vi "VALEW_Sensors_Arc.vi"(0 "GEA2 Reference In":refnum<k24>, 1 "Number of Pulses":i32=6, 2 "Expected Degree Change":u16=360, 5 "GEA Inputs":T1={"Source"=228, "Destination"=35} {"Destination" format="%.0x"; "Source" format="%.0x"}, 7 "DAQmx Physical Channel":tag="9401_1/ctr2", 9 "Counter Terminal":tag="/9401_1/PFI4", 11 "Error In":errorcluster, 14 "Standalone?":bool=TRUE) -> (4 "GEA2 Reference Out":refnum<k24>, 6 "Pass/Fail?":bool, 8 "Report Text":string, 10 "Actual Degree Change":u16, 15 "Error Out":errorcluster)   [LabVIEW 2016, in "TLMB.lvlib"]
doc: "This VI generates clock ticks on the hall sensor and ensures that they increase the arc sensor ERD appropriately. 8 Ticks should equal 360 degrees"
uses:
  Projects/TLMB.lvlib
  Q:/Common/DLLs/GEA3/GeaCommunication.dll
  Common/DLLs/GEA3/GeaCommunication.dll
  Common/LabVIEW GEA2 Toolkit/LabVIEW_GEA2_Toolkit.lvlibp/type defs/Source_Destination.ctl
  Common/LabVIEW GEA2 Toolkit/LabVIEW_GEA2_Toolkit.lvlibp/type defs/ERD Read Data In.ctl
  Common/LabVIEW GEA2 Toolkit/LabVIEW_GEA2_Toolkit.lvlibp/type defs/Data Type.ctl
  <vilib>/DAQmx/create/channels.llb/DAQmx Create Channel (CO-Pulse Generation-Frequency).vi
  <vilib>/DAQmx/configure/timing.llb/DAQmx Timing (Implicit).vi
  Common/LabVIEW GEA2 Toolkit/LabVIEW_GEA2_Toolkit.lvlibp
  <resource>/objmgr/daqmx.rc
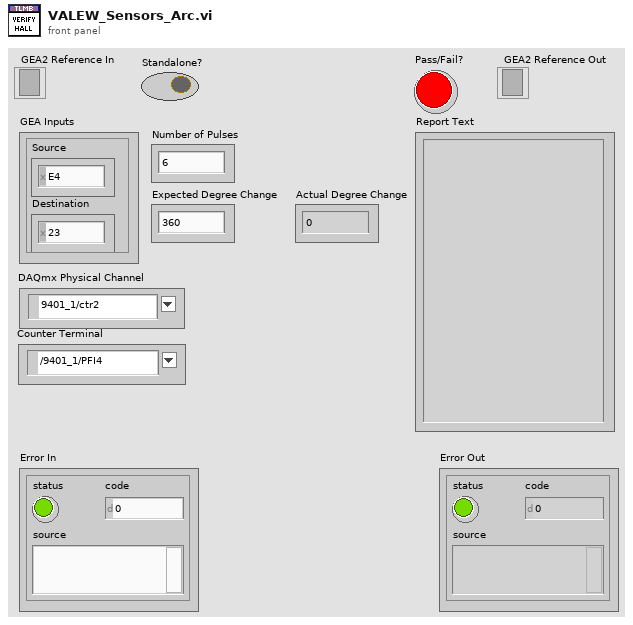
[diagram p1: front panel]
types:
  T1 = typedef "LabVIEW_GEA2_Toolkit.lvlibp/Source_Destination.ctl" = cluster{"Source":u8, "Destination":u8}
  T2 = typedef "LabVIEW_GEA2_Toolkit.lvlibp/ERD Read Data In.ctl" = cluster{"ERD Number":u16, "Data Type":T3}
  T3 = typedef "LabVIEW_GEA2_Toolkit.lvlibp/Data Type.ctl" = enum16{"string", "boolean", "uint8_t", "uint16_t", "uint32_t", "uint64_t", "int8_t", "int16_t", "int32_t", "int64_t"}
  T4 = typedef "LabVIEW_GEA2_Toolkit.lvlibp/ERD Read Data Out.ctl" = cluster{"ERD Number":u16, "Data":string}
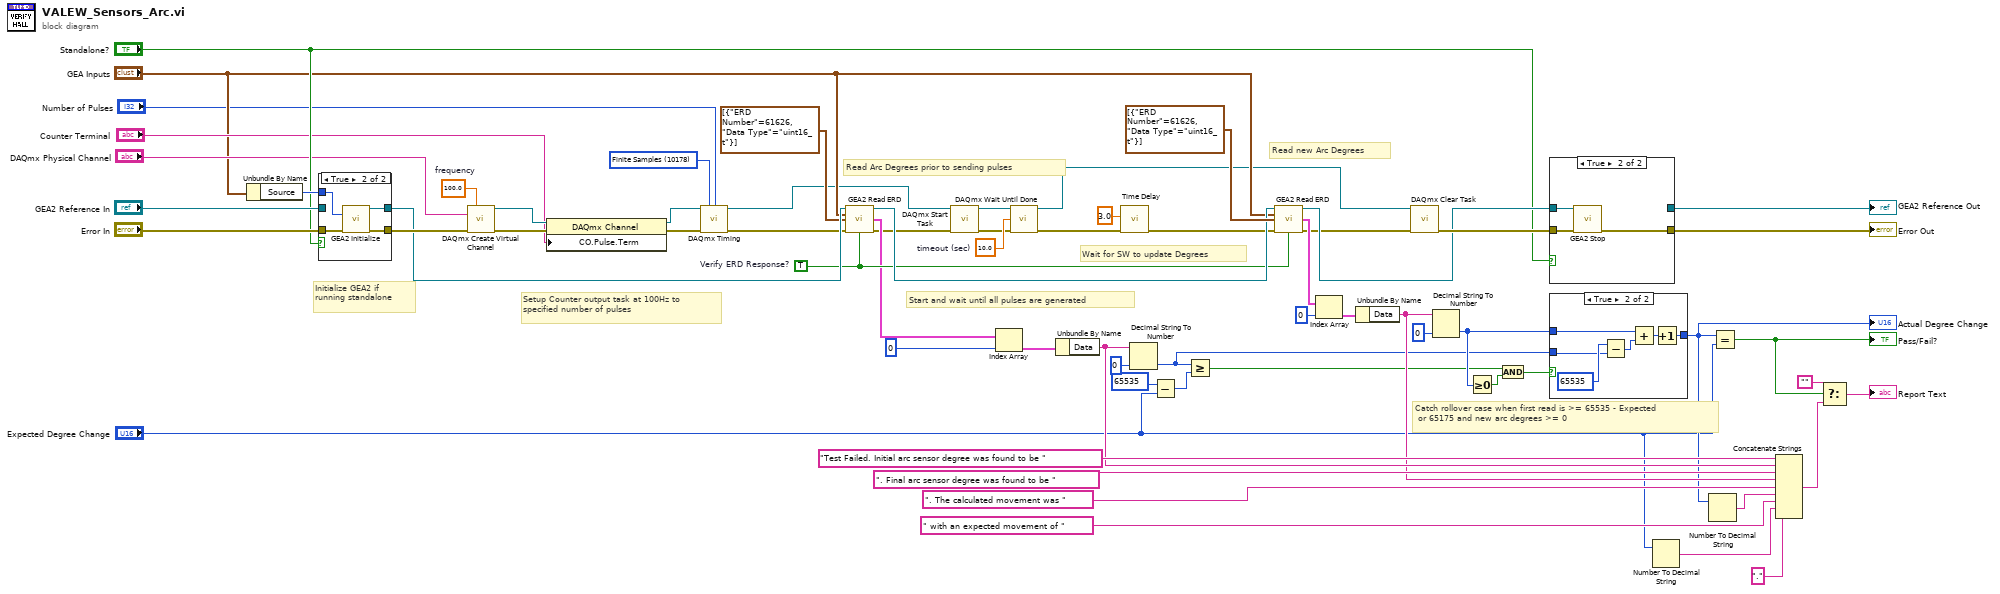
[diagram p0: block diagram]
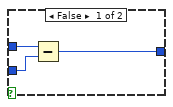
[diagram p2: hidden frame]
diagram:
  w34 = 10.0  # timeout (sec)
  w17 = 100.0  # frequency
  w41 = TRUE  # Verify ERD Response?
  w50 = 10178 items=["Finite Samples"=10178, "Continuous Samples"=10123, "Hardware Timed Single Point"=12522] ("sample mode")
  # "Catch rollover case when first read is >= 65535 - Expected\n or 65175 and new arc degrees >= 0"
  # "Read new Arc Degrees"
  # "Wait for SW to update Degrees"
  # "Start and wait until all pulses are generated"
  # "Read Arc Degrees prior to sending pulses"
  # "Setup Counter output task at 100Hz to\nspecified number of pulses"
  # "Initialize GEA2 if\nrunning standalone"
  n1 = Unbundle By Name("GEA Inputs") -> ("Source"=w58:u8)
  n2 = case shown="True" "Standalone?" {
    tunnel: "Error In" -> [w67 w71]
    tunnel: [w67 w70] -> w63
    tunnel: "GEA2 Reference In" -> [w66 _]
    tunnel: [w66 w69] -> w45
    tunnel: w58 -> [_ w68]
    frame False {
    }
    frame True {
      n3 = call "GEA2 Initialize.vi"("Source Address"=w68, "error in"=w71) -> ("GEA2 Reference Out"=w69:refnum<k24>, "error out"=w70:errorcluster)  [unwired: 11 in, 1 out]
    }
  }
  n4 = call-poly <vilib>:"DAQmx Create Virtual Channel.vi"("frequency"=w17, "counter"="DAQmx Physical Channel", "error in"=w63) -> ("task out"=w54:refnum<k21>, "error out"=w55:errorcluster)  [unwired: 11 in]
  n5 = property class="DAQmx Channel"(reference=w54, error in=w55, "CO.Pulse.Term"="Counter Terminal") -> (reference out=w51:refnum<k21>, error out=w14:errorcluster)
  n6 = call-poly <vilib>:"DAQmx Timing.vi"("task/channels in"=w51, "sample mode"=w50, "samples per channel"="Number of Pulses", "error in"=w14) -> ("task out"=w33:refnum<k21>, "error out"=w15:errorcluster)  [unwired: 10 in]
  n7 = call "GEA2 Read ERD.vi"("GEA2 Reference In"=w45, "GEA Inputs"="GEA Inputs", "Read ERD List"=T2[] [{"ERD Number"=61626, "Data Type"=enum."uint16_t"}], "Error In"=w15, "Verify ERD Response?"=w41) -> ("GEA2 Reference Out"=w44:refnum<k24>, "ERD Data Out"=w36:T4[], "Error Out"=w13:errorcluster)  [unwired: 7 in, 1 out]
  n8 = call <vilib>:"DAQmx Start Task.vi"("task/channels in"=w33, "error in"=w13) -> ("task out"=w11:refnum<k21>, "error out"=w12:errorcluster)  [unwired: 12 in]
  n9 = Index Array(array=w36, index=0) -> (element=w37:T4)
  n10 = call <vilib>:"DAQmx Wait Until Done.vi"("task/channels in"=w11, "timeout (sec)"=w34, "error in"=w12) -> ("task out"=w35:refnum<k21>, "error out"=w10:errorcluster)  [unwired: 11 in]
  n11 = Unbundle By Name(w37) -> ("Data"=w28:string)
  n12 = call "Time Delay"("error in (no error)"=w10, "Delay Time (s)"=3.0) -> ("error out"=w9:errorcluster)  [unwired: 9 in]
  n13 = Decimal String To Number(string=w28, default (0L)=u16 0 ("default (0 I32)")) -> (number=w2:u16)  [unwired: 1 in, 1 out]
  n14 = Subtract(x=u16 65535, y="Expected Degree Change") -> (x-y=w1:u16)
  n15 = Greater Or Equal?(x=w2, y=w1) -> (x >= y?=w7:bool)
  n16 = call "GEA2 Read ERD.vi"("GEA2 Reference In"=w44, "GEA Inputs"="GEA Inputs", "Read ERD List"=T2[] [{"ERD Number"=61626, "Data Type"=enum."uint16_t"}], "Error In"=w9, "Verify ERD Response?"=w41) -> ("GEA2 Reference Out"=w59:refnum<k24>, "ERD Data Out"=w49:T4[], "Error Out"=w32:errorcluster)  [unwired: 7 in, 1 out]
  n17 = Index Array(array=w49, index=0) -> (element=w47:T4)
  n18 = Unbundle By Name(w47) -> ("Data"=w26:string)
  n19 = call <vilib>:"DAQmx Clear Task.vi"("task in"=w35, "error in"=w32) -> ("error out"=w62:errorcluster)  [unwired: 13 in]
  n20 = Decimal String To Number(string=w26, default (0L)=u16 0 ("default (0 I32)")) -> (number=w8:u16)  [unwired: 1 in, 1 out]
  n21 = Greater Or Equal To 0?(x=w8) -> (x >= 0?=w6:bool)
  n22 = And(x=w7, y=w6) -> (x .and. y?=w5:bool)
  n23 = case shown="True" "Standalone?" {
    tunnel: [w72 w76] -> w60
    tunnel: w59 -> [w73 w74]
    tunnel: [w73 _] -> w61
    tunnel: w62 -> [w72 w75]
    frame False {
    }
    frame True {
      n24 = call "GEA2 Stop.vi"("GEA2 Reference In"=w74, "Error In"=w75) -> ("Error Out"=w76:errorcluster)  [unwired: 13 in]
    }
  }
  "Error Out" <- w60
  "GEA2 Reference Out" <- w61
  n25 = case shown="True" w5 {
    tunnel: w2 -> [w79 w84]
    tunnel: w8 -> [w78 w82]
    tunnel: [w77 w81] -> w24
    frame False {
      n26 = Subtract(x=w78, y=w79) -> (x-y=w77:u16)
    }
    frame True {
      n27 = Subtract(x=u16 65535, y=w84) -> (x-y=w83:u16)
      n28 = Add(x=w82, y=w83) -> (x+y=w80:u16)
      n29 = Increment(x=w80) -> (x+1=w81:u16)
    }
  }
  "Actual Degree Change" <- w24
  n30 = Number To Decimal String(number="Expected Degree Change") -> (decimal integer string=w21:string)  [unwired: 1 in]
  n31 = Number To Decimal String(number=w24) -> (decimal integer string=w23:string)  [unwired: 1 in]
  n32 = Equal?(x=w24, y="Expected Degree Change") -> (x = y?=w31:bool)
  "Pass/Fail?" <- w31
  n33 = Concatenate Strings("Test Failed. Initial arc sensor degree was found to be ", w28, ". Final arc sensor degree was found to be ", w26, ". The calculated movement was " ("string"), w23, " with an expected movement of " ("string"), w21, "." ("string")) -> (w19:string)
  n34 = Select(t="", s=w31, f=w19) -> (s? t:f=→"Report Text":string)
